vi "RPM 600 速度轉電壓 三軸平台 Axis 1.vi"(1 "Speed (1mm/s)":dbl) -> (0 "Voltage\nOutput":dbl)   [LabVIEW 2019]
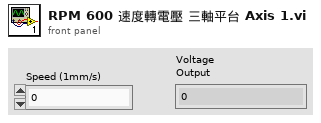
[diagram p1: front panel]
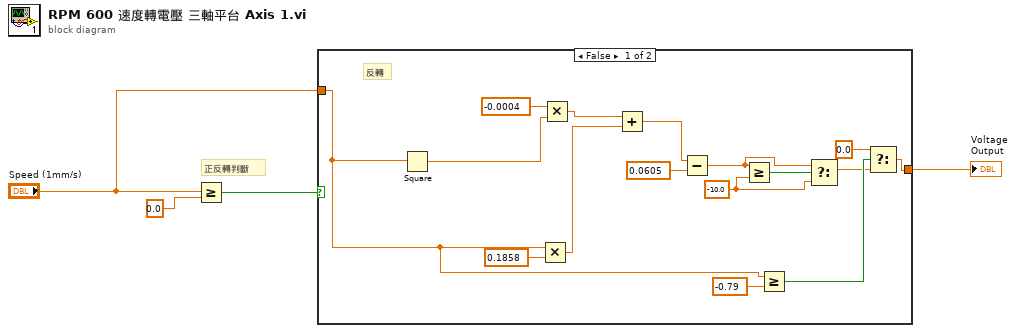
[diagram p0: block diagram]
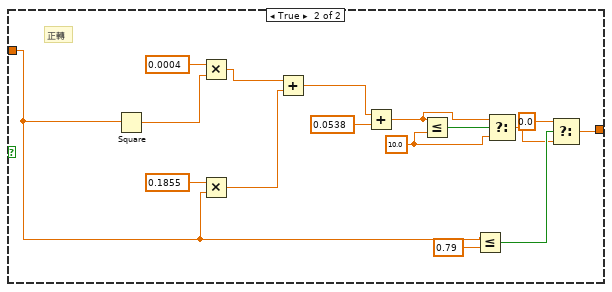
[diagram p2: hidden frame]
diagram:
  # "正反轉判斷"
  n1 = Greater Or Equal?(x="Speed (1mm/s)", y=0.0) -> (x >= y?=w3:bool)
  n2 = case shown="False" w3 {
    tunnel: "Speed (1mm/s)" -> [w9 w26]
    tunnel: [w5 w24] -> w1
    frame False {
      w14 = -10.0 ("y")
      # "反轉"
      n3 = Square(x=w9) -> (x^2=w20:dbl)
      n4 = Multiply(x=w9, y=0.1858) -> (x*y=w16:dbl)
      n5 = Multiply(x=-0.0004, y=w20) -> (x*y=w19:dbl)
      n6 = Add(x=w19, y=w16) -> (x+y=w18:dbl)
      n7 = Subtract(x=w18, y=0.0605) -> (x-y=w13:dbl)
      n8 = Greater Or Equal?(x=w13, y=w14) -> (x >= y?=w15:bool)
      n9 = Greater Or Equal?(x=w9, y=-0.79) -> (x >= y?=w8:bool)
      n10 = Select(t=w13, s=w15, f=w14) -> (s? t:f=w6:dbl)
      n11 = Select(t=0.0, s=w8, f=w6) -> (s? t:f=w5:dbl)
    }
    frame True {
      w30 = 10.0 ("y")
      # "正轉"
      n12 = Square(x=w26) -> (x^2=w36:dbl)
      n13 = Multiply(x=0.0004, y=w36) -> (x*y=w35:dbl)
      n14 = Multiply(x=0.1855, y=w26) -> (x*y=w34:dbl)
      n15 = Add(x=w35, y=w34) -> (x+y=w33:dbl)
      n16 = Add(x=w33, y=0.0538) -> (x+y=w29:dbl)
      n17 = Less Or Equal?(x=w29, y=w30) -> (x <= y?=w31:bool)
      n18 = Less Or Equal?(x=w26, y=0.79) -> (x <= y?=w23:bool)
      n19 = Select(t=w29, s=w31, f=w30) -> (s? t:f=w22:dbl)
      n20 = Select(t=0.0, s=w23, f=w22) -> (s? t:f=w24:dbl)
    }
  }
  "Voltage\nOutput" <- w1
